vi "Split 1D ARRAY in half.vi"(11 "Array in":dbl[](array[numeric])) -> (2 "Array out":dbl[](array[numeric]), 3 "Array 3":dbl[](array[numeric]))   [LabVIEW 2016, in "Instrument.Lockin.lvclass"]
uses:
  Instrument.Lockin.lvclass
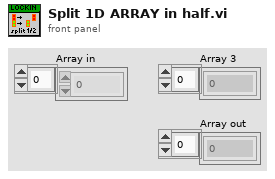
[diagram p1: front panel]
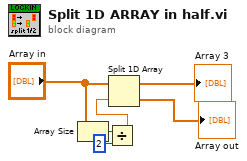
[diagram p0: block diagram]
diagram:
  n1 = Array Size(array="Array in") -> (size(s)=w4:i32)
  n2 = Divide(x=w4, y=2) -> (x/y=w5:dbl)
  n3 = Split 1D Array(array="Array in", index=w5) -> (first subarray=→"Array 3":dbl[], second subarray=→"Array out":dbl[])
